vi "Get Websocket Info.vi"(8 "error in (no error)":errorcluster) -> (0 "error out":errorcluster, 3 "Connection Info":T1)   [LabVIEW 2015, in "Front Panel Publisher.lvlib" / "Front Panel Manager.lvclass"]
uses:
  Front Panel Manager.lvclass
  Controls/Websocket Info.ctl
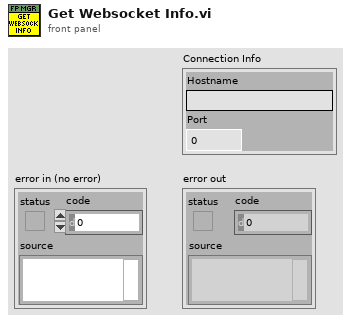
[diagram p1: front panel]
types:
  T1 = typedef "Front Panel Publisher.lvlib/Front Panel Manager.lvclass/Websocket Info.ctl" = cluster{"Hostname":string, "Port":u16}
  T2 = typedef "Front Panel Publisher.lvlib/Front Panel Manager.lvclass/Object Attributes.ctl" = cluster{"WebFrontPanels":refnum<class "Web Front Panel.lvclass">[], "WFP Names":string[], "Root folder":path, "Websocket Info":T1}
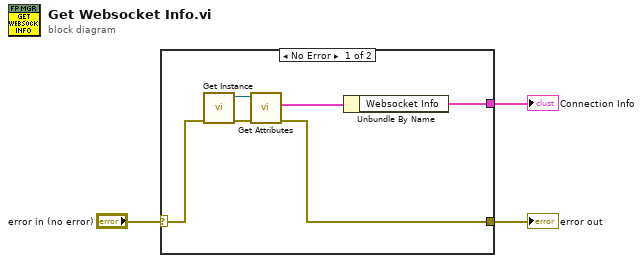
[diagram p0: block diagram]
diagram:
  n1 = case shown="No Error" "error in (no error)" {
    selector: "error in (no error)" -> [w5 w10]
    tunnel: [w8 w10] -> w2
    tunnel: [w7 _] -> w1
    frame No Error {
      n2 = call "Get Instance.vi"("error in (no error)"=w5) -> ("error out"=w4:errorcluster, "FP Manager Out"=w6:refnum<class "Front Panel Manager.lvclass">)  [unwired: 6 in, 3 out]
      n3 = call "Get Attributes.vi"("error in (no error)"=w4, "FP Management In"=w6) -> ("error out"=w8:errorcluster, "Data"=w9:T2)  [unwired: 6 in, 2 out]
      n4 = Unbundle By Name(w9) -> ("Websocket Info"=w7:T1)
    }
    frame Error {
    }
  }
  "error out" <- w2
  "Connection Info" <- w1
